vi "AlliGator FMB Check for Abort.vi"(1 "Named Q Elements":T1[](array[typedef])) -> (0 "Named Q Elements":T1[](array[typedef]))   [LabVIEW 2021, in "AlliGator Fit Method Benchmark.lvlib"]
uses:
  AlliGator Fit Method Benchmark.lvlib
  AlliGator FMB Q Element.ctl
  AlliGator FMB Q Event List.ctl
panel:
  # "see the License on the block diagram (Ctrl+E or Window:Show Block Diagram)"
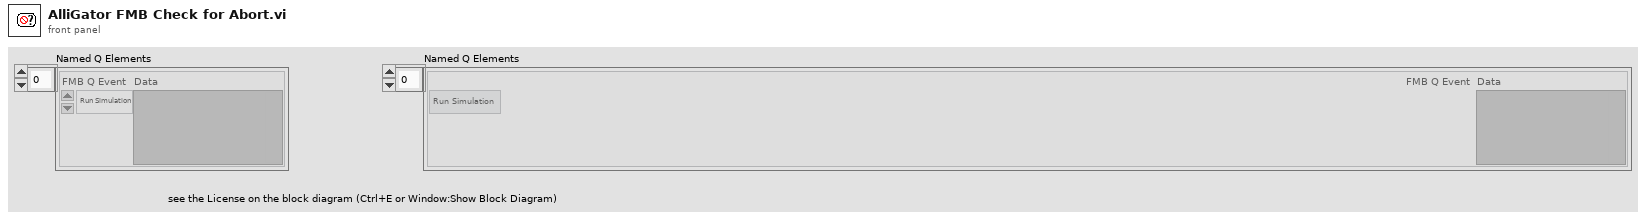
[diagram p1: front panel]
types:
  T1 = typedef "AlliGator Fit Method Benchmark.lvlib/AlliGator FMB Q Element.ctl" = cluster{"FMB Q Event":T2, "Data":variant}
  T2 = typedef "AlliGator Fit Method Benchmark.lvlib/AlliGator FMB Q Event List.ctl" = enum16{"Idle", "Initialization", "Update Script Simulation Parameters", "Single Simulation Prelude", "Run Simulation", "Update Histograms", "Update Script Simulation Output", "Graph Event", "Show Selected Decay", "Export Results", "Update # Processors Used", "Check Baseline", "Run Script", "End Script", "Init", "Abort", "Quit"}
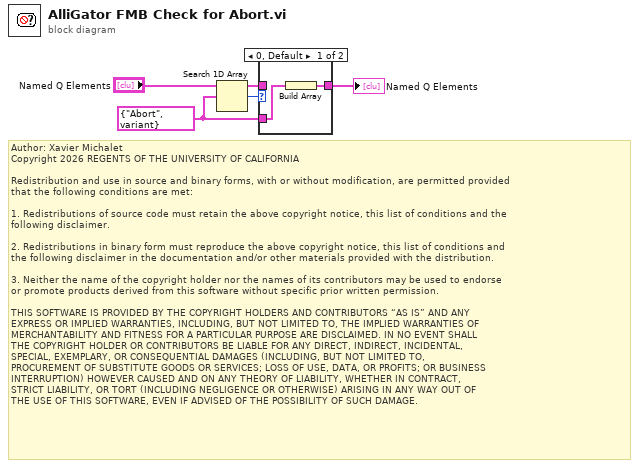
[diagram p0: block diagram]
diagram:
  w1 = T1 {"FMB Q Event"=enum."Abort", "Data"=variant} ("element")
  # "Author: Xavier Michalet\nCopyright 2026 REGENTS OF THE UNIVERSITY OF CALIFORNIA\n\nRedistribution and use in source and binary forms, with or without modification, are permitted provided\nthat the following conditions are met:\n\n1. Redistributions of source code must retain the above copyright notice, this list of conditions and the\nfollowing disclaimer.\n\n2. Redistributions in binary form must reproduce the above copyright notice, this list of conditions and\nthe following disclaimer in the documentation and/or other materials provided with the distribution.\n\n3. Neither the name of the copyright holder nor the names of its contributors may be used to endorse \nor promote products derived from this software without specific prior written permission.\n\nTHIS SOFTWARE IS PROVIDED BY THE COPYRIGHT HOLDERS AND CONTRIBUTORS “AS IS” AND ANY \nEXPRESS OR IMPLIED WARRANTIES, INCLUDING, BUT NOT LIMITED TO, THE IMPLIED WARRANTIES OF\nMERCHANTABILITY AND FITNESS FOR A PARTICULAR PURPOSE ARE DISCLAIMED. IN NO EVENT SHALL\nTHE COPYRIGHT HOLDER OR CONTRIBUTORS BE LIABLE FOR ANY DIRECT, INDIRECT, INCIDENTAL, \nSPECIAL, EXEMPLARY, OR CONSEQUENTIAL DAMAGES (INCLUDING, BUT NOT LIMITED TO, \nPROCUREMENT OF SUBSTITUTE GOODS OR SERVICES; LOSS OF USE, DATA, OR PROFITS; OR BUSINESS\nINTERRUPTION) HOWEVER CAUSED AND ON ANY THEORY OF LIABILITY, WHETHER IN CONTRACT, \nSTRICT LIABILITY, OR TORT (INCLUDING NEGLIGENCE OR OTHERWISE) ARISING IN ANY WAY OUT OF\nTHE USE OF THIS SOFTWARE, EVEN IF ADVISED OF THE POSSIBILITY OF SUCH DAMAGE."
  n1 = Search 1D Array(1D array="Named Q Elements", element=w1) -> (index of element=w4:i32)  [unwired: 1 in]
  n2 = case shown="0, Default" w4 {
    tunnel: "Named Q Elements" -> [_ w7]
    tunnel: [w5 w7] -> w2
    tunnel: w1 -> [w6 _]
    frame 0, Default {
      n3 = Build Array(w6) -> (w5:T1[])
    }
    frame -1 {
    }
  }
  "Named Q Elements" <- w2
